vi "Subtract Months From Timestamp.vi"(10 "Months":i32=12, 11 "Start Time":timestamp) -> (3 "End Time":timestamp)   [LabVIEW 2011]
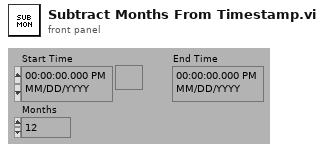
[diagram p1: front panel]
types:
  T1 = typedef "LVDateTimeRec.ctl" = cluster{"fractional second":dbl, "second":i32, "minute":i32, "hour":i32, "day of month":i32, "month":i32, "year":i32, "day of week":i32, "day of year":i32, "DST":i32}
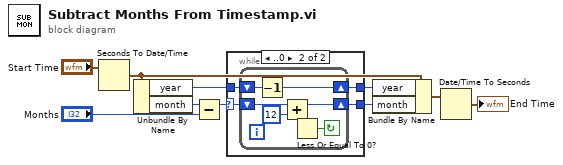
[diagram p0: block diagram]
diagram:
  n1 = Seconds To Date/Time(time stamp (now)="Start Time") -> (date time rec=w10:T1)  [unwired: 1 in]
  n2 = Unbundle By Name(w10) -> ("year"=w3:i32, "month"=w6:i32)
  n3 = Subtract(x=w6, y="Months") -> (x-y=w4:i32)
  n4 = case shown="..0" w4 {
    selector: w4 -> [w11 w16]
    tunnel: w3 -> [w12 w15]
    tunnel: [w11 w14] -> w2
    tunnel: [w12 w13] -> w1
    frame Default {
    }
    frame ..0 {
      n5 = while {
        shift-right: [w20] -> w13
        shift-left: w15 -> [w21]
        shift-right: [w17] -> w14
        shift-left: w16 -> [w19]
        stop <- w22 continue-if-true
        n6 = Decrement(x=w21) -> (x-1=w20:i32)
        n7 = Add(x=w19, y=12) -> (x+y=w17:i32)
        n8 = Less Or Equal To 0?(x=w17) -> (x <= 0?=w22:bool)
      }
    }
  }
  n9 = Bundle By Name(cluster=w10, "year"=w1, "month"=w2) -> (w8:T1)
  n10 = Date/Time To Seconds(2:w8) -> (0:→"End Time":timestamp)  [unwired: 1 in]
